vi "plusminusU8.vi"(5 "y":u8, 6 "x":u8) -> (1 "x - y":u8, 2 "x + y":u8)   [LabVIEW 2017]
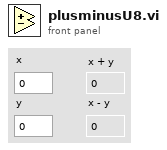
[diagram p1: front panel]
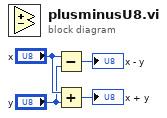
[diagram p0: block diagram]
diagram:
  n1 = Subtract(x="x", y="y") -> (x-y=→"x - y":u8)
  n2 = Add(x="x", y="y") -> (x+y=→"x + y":u8)
